vi "TelemetryDev.vi"(8 "error in":errorcluster, 10 "ON/OFF":bool, 11 "VISA resource name in":refnum<visa-resource-name>) -> (0 "error out":errorcluster, 3 "VISA resource name out":refnum<visa-resource-name>, 4 "Laser PRR, kHz":dbl caption="Частота следования импульсов" format="%#_g kHz", 6 "module temp":dbl caption="Темп. модуля" format="%#_g °C", 7 "Laser Power,%":dbl caption="Мощьность, %" format="%#_g ")   [LabVIEW 2014]
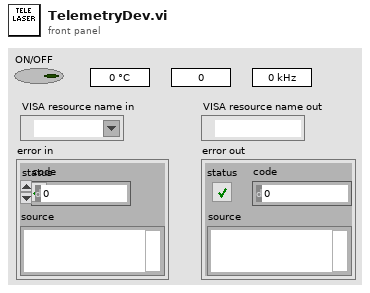
[diagram p1: front panel]
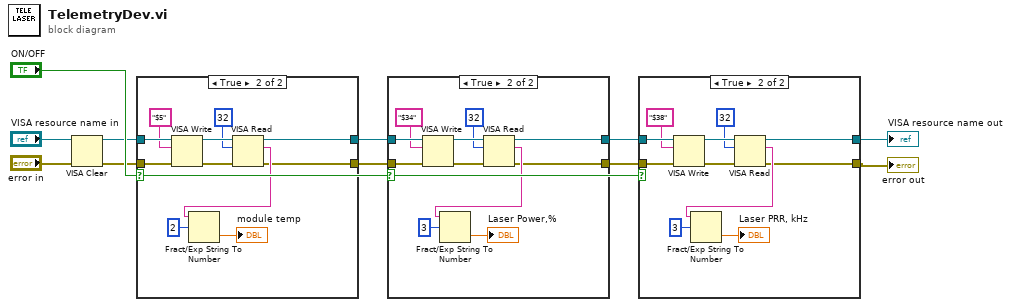
[diagram p0: block diagram]
diagram:
  n1 = VISA Clear(VISA resource name="VISA resource name in", error in (no error)="error in") -> (VISA resource name out=w4:refnum<visa-resource-name>, error out=w3:errorcluster)
  n2 = case shown="True" "ON/OFF" {
    tunnel: w4 -> [w13 w22]
    tunnel: w3 -> [w12 w21]
    tunnel: [w13 w15] -> w11
    tunnel: [w12 w14] -> w10
    frame False {
    }
    frame True {
      n3 = VISA Write(VISA resource name=w22, write buffer="$5", error in (no error)=w21) -> (VISA resource name out=w23:refnum<visa-resource-name>, error out=w24:errorcluster)  [unwired: 1 out]
      n4 = VISA Read(VISA resource name=w23, byte count=u32 32, error in (no error)=w24) -> (VISA resource name out=w15:refnum<visa-resource-name>, read buffer=w18:string, error out=w14:errorcluster)  [unwired: 1 out]
      n5 = Fract/Exp String To Number(string=w18, offset=2) -> (number=→"module temp":dbl)  [unwired: 2 in, 1 out]
    }
  }
  n6 = case shown="True" "ON/OFF" {
    tunnel: w11 -> [w26 w35]
    tunnel: w10 -> [w25 w34]
    tunnel: [w26 w28] -> w7
    tunnel: [w25 w27] -> w6
    frame False {
    }
    frame True {
      n7 = VISA Write(VISA resource name=w35, write buffer="$34", error in (no error)=w34) -> (VISA resource name out=w36:refnum<visa-resource-name>, error out=w37:errorcluster)  [unwired: 1 out]
      n8 = VISA Read(VISA resource name=w36, byte count=u32 32, error in (no error)=w37) -> (VISA resource name out=w28:refnum<visa-resource-name>, read buffer=w31:string, error out=w27:errorcluster)  [unwired: 1 out]
      n9 = Fract/Exp String To Number(string=w31, offset=3) -> (number=→"Laser Power,%":dbl)  [unwired: 2 in, 1 out]
    }
  }
  n10 = case shown="True" "ON/OFF" {
    tunnel: w7 -> [w39 w48]
    tunnel: w6 -> [w38 w47]
    tunnel: [w39 w41] -> w9
    tunnel: [w38 w40] -> w8
    frame False {
    }
    frame True {
      n11 = VISA Write(VISA resource name=w48, write buffer="$38", error in (no error)=w47) -> (VISA resource name out=w49:refnum<visa-resource-name>, error out=w50:errorcluster)  [unwired: 1 out]
      n12 = VISA Read(VISA resource name=w49, byte count=u32 32, error in (no error)=w50) -> (VISA resource name out=w41:refnum<visa-resource-name>, read buffer=w44:string, error out=w40:errorcluster)  [unwired: 1 out]
      n13 = Fract/Exp String To Number(string=w44, offset=3) -> (number=→"Laser PRR, kHz":dbl)  [unwired: 2 in, 1 out]
    }
  }
  "VISA resource name out" <- w9
  "error out" <- w8
